vi "Read Current Sense Resistivity.vi"(8 "error in (no error)":errorcluster, 11 "configuration file path":path) -> (0 "error out":errorcluster, 2 "Array":dbl[](array[numeric]), 3 "file path":path)   [LabVIEW 2023]
uses:
  <vilib>/Utility/config.llb/Read Key (Double).vi
  <vilib>/Utility/config.llb/NI_LVConfig.lvlib
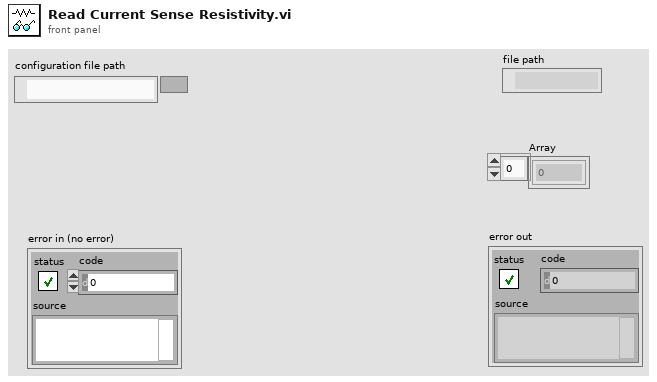
[diagram p1: front panel]
types:
  T1 = typedef "NI_LVConfig.lvlib/Config Data RefNum.ctl" = refnum<k1>
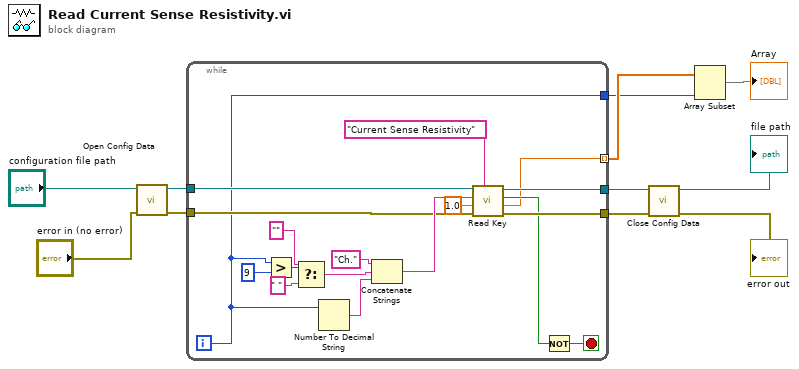
[diagram p0: block diagram]
diagram:
  n1 = call <vilib>:"Open Config Data.vi"("error in (no error)"="error in (no error)", "configuration file path"="configuration file path") -> ("error out"=w7:errorcluster, "refnum"=w6:T1)  [unwired: 7 in, 1 out]
  n2 = while {
    tunnel: [w28] -> w11
    tunnel: [w27] -> w10
    tunnel: [w21] -> w3 mode=indexing
    tunnel: w7 -> [w20]
    tunnel: w6 -> [w19]
    tunnel: [w12] -> w1
    i -> [w12]
    stop <- w22 stop-if-true
    n3 = Greater?(x=w12, y=9) -> (0:w16:bool)
    n4 = Select(t="" ("string"), s=w16, f=" " ("string")) -> (s? t:f=w13:string)
    n5 = Number To Decimal String(number=w12) -> (decimal integer string=w26:string)  [unwired: 1 in]
    n6 = Concatenate Strings("Ch." ("string"), w13, w26) -> (w25:string)
    n7 = call-poly <vilib>:"Read Key.vi"("section"="Current Sense Resistivity", "error in (no error)"=w20, "default value"=1.0, "key"=w25, "refnum"=w19) -> ("error out"=w27:errorcluster, "value"=w21:dbl, "found?"=w23:bool, "refnum out"=w28:T1)  [unwired: 3 in]
    n8 = Not(x=w23) -> (.not. x?=w22:bool)
  }
  n9 = call <vilib>:"Close Config Data.vi"("error in (no error)"=w10, "refnum"=w11) -> ("error out"=→"error out":errorcluster, "file path"=→"file path":path)  [unwired: 8 in]
  n10 = Array Subset(array=w3, length=w1) -> (→"Array":dbl[])  [unwired: 1 in]
